vi "Release Logger.vi"(8 "error in (no error)":errorcluster, 11 "Log Producer in":T1) -> (0 "error out":errorcluster, 3 "Log Producer out":T1)   [LabVIEW 2020, in "Frame Logging.lvlib"]
uses:
  Frame Logging.lvlib
  Message_Request_Action.ctl
  Message_Request.ctl
  Log_Producer.ctl
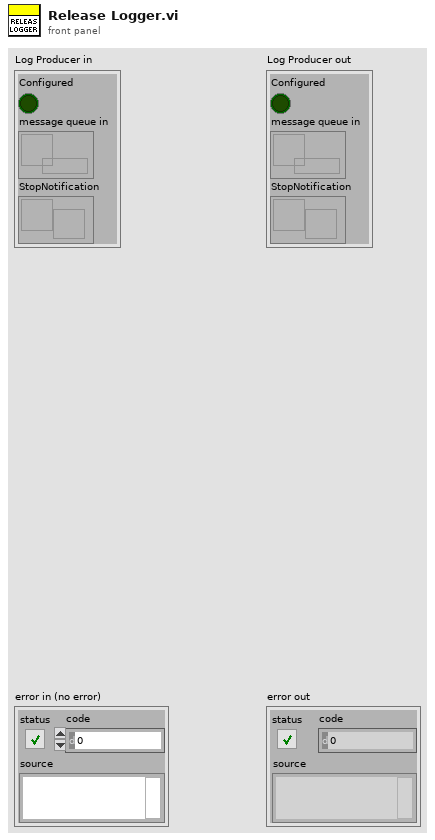
[diagram p1: front panel]
types:
  T1 = typedef "Frame Logging.lvlib/Log_Producer.ctl" = cluster{"Configured":bool, "message queue in":refnum<queue>, "StopNotification":refnum<notifier>}
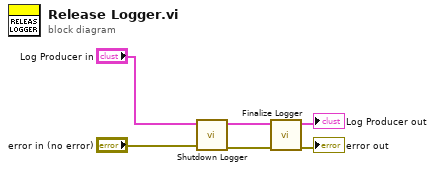
[diagram p0: block diagram]
diagram:
  n1 = call "Shutdown Logger.vi"("error in"="error in (no error)", "Log Producer in"="Log Producer in") -> ("error out"=w2:errorcluster, "Log Producer out"=w1:T1)  [unwired: 8 in]
  n2 = call "Finalize Logger.vi"("error in"=w2, "Log Producer in"=w1) -> ("error out"=→"error out":errorcluster, "Log Producer out"=→"Log Producer out":T1)  [unwired: 8 in]
